vi "FRCts20_Backend_Test_TeamRoot_GET.vi"(8 "error in (no error)":errorcluster) -> (0 "error out":errorcluster, 1 "Time (ms)":u32, 2 "Status":string, 3 "Team Out":T1, 5 "Success":bool)   [LabVIEW 2014, in "FRCts20_Backend_TestCode.lvlib"]
uses:
  FRCts20_Backend_TestCode.lvlib
  FRCts20_Backend_API/FRCts20_Backend_API_Command_TeamRoot.ctl
  FRCts20_Backend_API/FRCts20_Backend_API_SW.ctl
  FRCts20_Backend_API/FRCts20_Backend_API_TeamRoot.ctl
  FRCts20_Backend_API/FRCts20_Backend_API_TeamRoot.vi
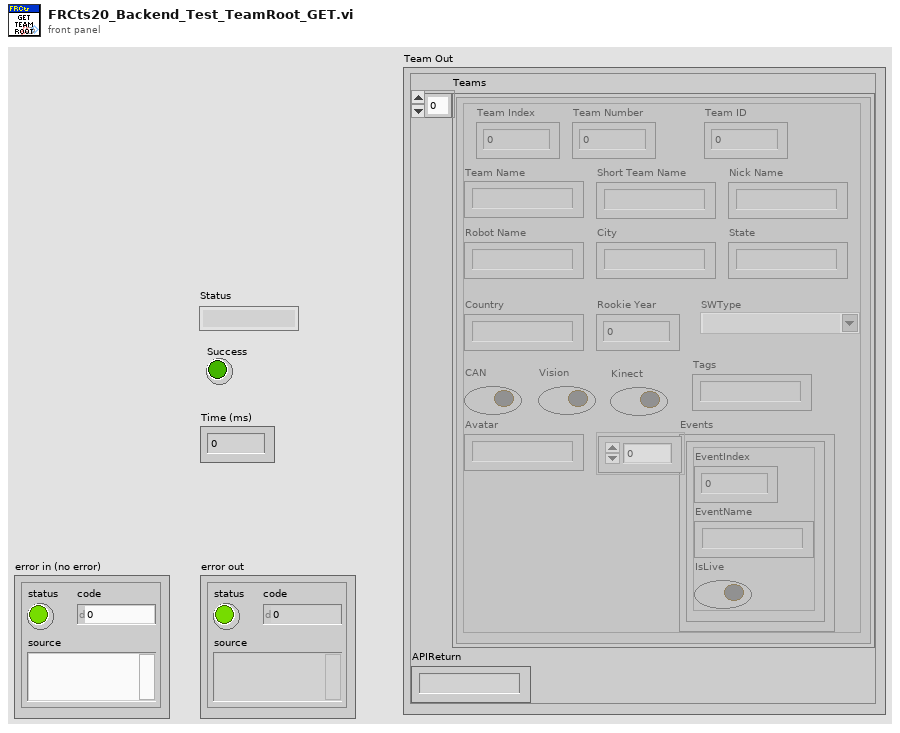
[diagram p1: front panel]
types:
  T1 = typedef "FRCts20_Backend_API.lvlib/FRCts20_Backend_API_TeamRoot.ctl" = cluster{"Teams":cluster{"Team Index":u32, "Team Number":u32, "Team ID":u32, "Team Name":string, "Short Team Name":string, "Nick Name":string, "Robot Name":string, "City":string, "State":string, "Country":string, "Rookie Year":u32, "SWType":T2, "CAN":bool, "Vision":bool, "Kinect":bool, "Tags":string, "Avatar":string, "Events":cluster{"EventIndex":u32, "EventName":string, "IsLive":bool}[]}[], "APIReturn":string}
  T2 = typedef "FRCts20_Backend_API.lvlib/FRCts20_Backend_API_SW.ctl" = string
  T3 = typedef "FRCts20_Backend_API.lvlib/FRCts20_Backend_API_Command_TeamRoot.ctl" = string
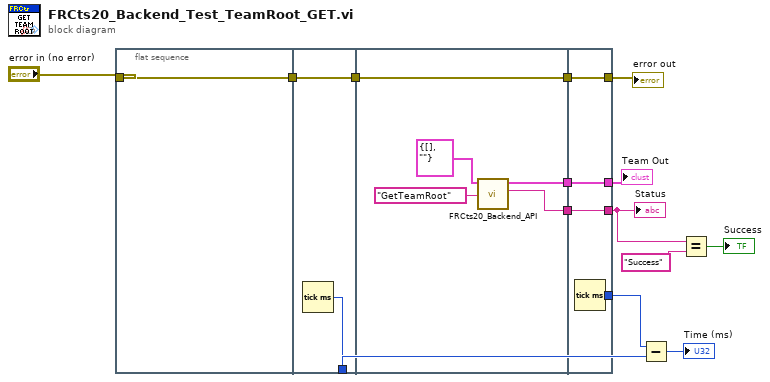
[diagram p0: block diagram]
diagram:
  n1 = flat-sequence {
    tunnel: "error in (no error)" -> [w15]
    tunnel: [w15] -> w14
    tunnel: [w17] -> w4
    tunnel: [w16] -> w13
    tunnel: w14 -> [w16]
    tunnel: [w22] -> w12
    tunnel: w13 -> [w22]
    tunnel: [w20] -> w11
    tunnel: [w19] -> w2
    tunnel: [w26] -> w5
    tunnel: [w25] -> w7
    tunnel: w12 -> [w25]
    tunnel: [w24] -> w3
    tunnel: w11 -> [w24]
    tunnel: [w23] -> w1
    tunnel: w2 -> [w23]
    frame #0 {
    }
    frame #1 {
      n2 = Tick Count (ms)() -> (millisecond timer value=w17:u32)
    }
    frame #2 {
      n3 = call-poly "FRCts20_Backend_API.vi"("Command"=T3 "GetTeamRoot", "Team In"=T1 {"Teams"=[], "APIReturn"=""}) -> ("Status"=w20:string, "Team Out"=w19:T1)  [unwired: 7 in, 1 out]
    }
    frame #3 {
      n4 = Tick Count (ms)() -> (millisecond timer value=w26:u32)
    }
  }
  n5 = Subtract(x=w5, y=w4) -> (x-y=→"Time (ms)":u32)
  n6 = Equal?(x=w3, y="Success") -> (x = y?=→"Success":bool)
  "Status" <- w3
  "error out" <- w7
  "Team Out" <- w1
